vi "confirm_ast.vi"(11 "ImgAstrom IN":T1 {"CRVAL" format="%.6g"; "CD" format="%_7g"}) -> (0 "Accepted?":bool, 3 "ImgAstrom OUT":T1 {"CRVAL" format="%.6g"; "CD" format="%_7g"})   [LabVIEW 2019]
panel:
  in  "refuse":bool
  in  "Accept":bool
  # "Confirmer que les données astrométriques\nprésentées ci-dessous sont bonnes ..."
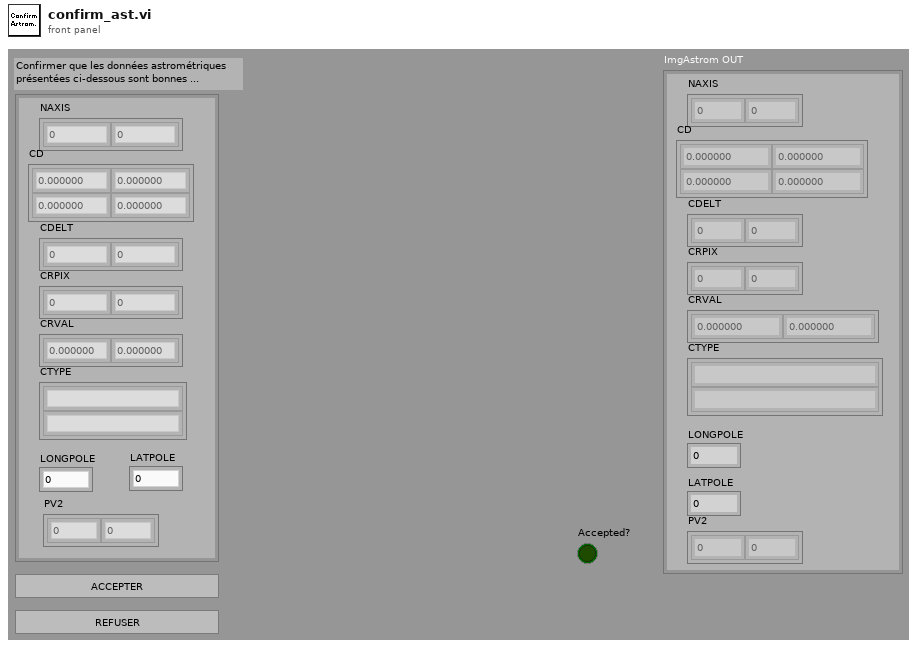
[diagram p1: front panel]
types:
  T1 = cluster{"NAXIS":dbl[], "CD":dbl[][], "CDELT":dbl[], "CRPIX":dbl[], "CTYPE":string[], "CRVAL":dbl[], "LONGPOLE":dbl, "LATPOLE":dbl, "PV2":dbl[]}
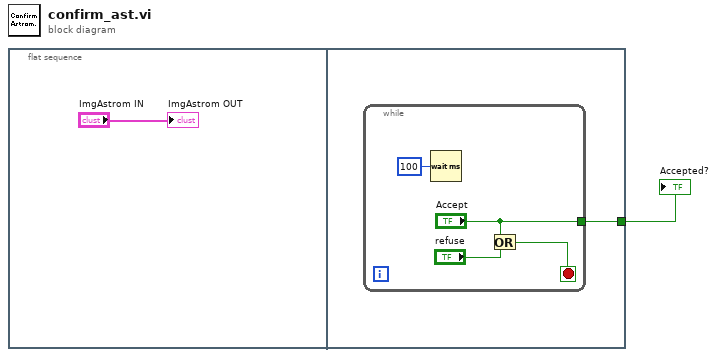
[diagram p0: block diagram]
diagram:
  n1 = flat-sequence {
    tunnel: [w3] -> w1
    frame #0 {
      "ImgAstrom OUT" <- "ImgAstrom IN"
    }
    frame #1 {
      n2 = while {
        tunnel: ["Accept"] -> w3
        stop <- w5 stop-if-true
        n3 = Wait (ms)(milliseconds to wait=u32 100) -> ()  [unwired: 1 out]
        n4 = Or(x="Accept", y="refuse") -> (x .or. y?=w5:bool)
      }
    }
  }
  "Accepted?" <- w1
